vi "RS232test.vi"() -> ()   [LabVIEW 2014]
panel:
  out "Tweet text":string
  in  "Send Tweets?":bool
  out "Run Time (s)":dbl
  out "CTS?":bool
  out "DSR?":bool
  out "Serial Settings:Modem Line Settings:Line DSR State":i16(ring)=-1 items=["Unknown"=-1, "Unasserted"=0, "Asserted"=1]
  out "Serial Settings:Modem Line Settings:Line CTS State":i16(ring)=-1 items=["Unknown"=-1, "Unasserted"=0, "Asserted"=1]
  out "error out":errorcluster
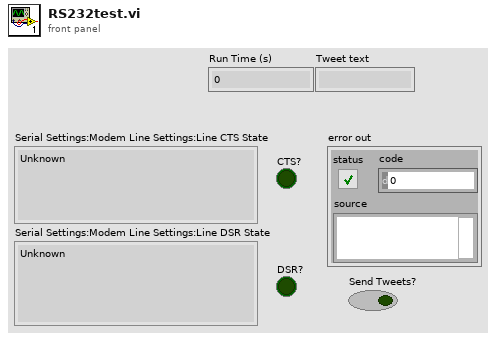
[diagram p1: front panel]
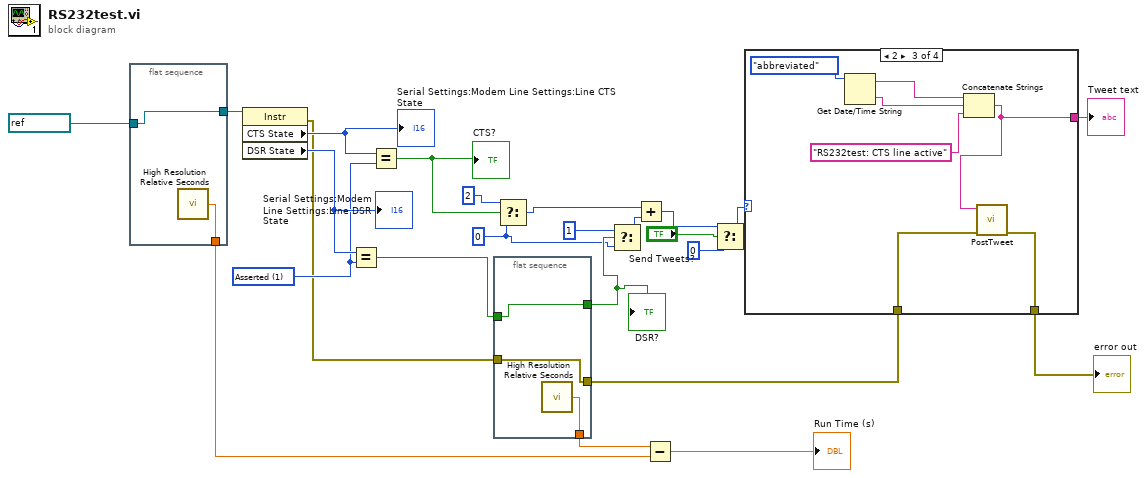
[diagram p0: block diagram]
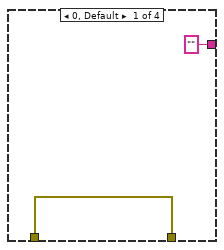
[diagram p2: hidden frame]
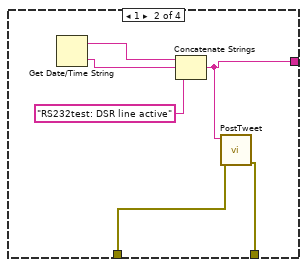
[diagram p3: hidden frame]
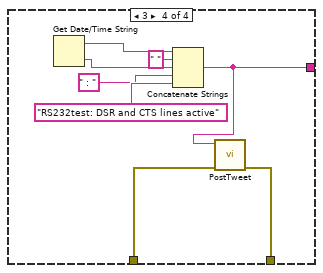
[diagram p4: hidden frame]
diagram:
  w9 = u8 0 ("f")
  w22 = i16 1 items=["Unknown"=-1, "Unasserted"=0, "Asserted"=1] ("Serial Settings:Modem Line Settings:Line DSR State 2")
  n1 = flat-sequence {
    tunnel: refnum<visa-resource-name> "COM1" ("VISA resource name") -> [w26]
    tunnel: [w26] -> w20
    tunnel: [w25] -> w17
    frame #0 {
      n2 = call <vilib>:"High Resolution Relative Seconds.vi"() -> ("relative seconds"=w25:dbl)
    }
  }
  n3 = property class="Instr"(reference=w20) -> (error out=w15:errorcluster, "CTS State"=w23:i16, "DSR State"=w24:i16)  [unwired: 1 in, 1 out]
  "Serial Settings:Modem Line Settings:Line CTS State" <- w23
  "Serial Settings:Modem Line Settings:Line DSR State" <- w24
  n4 = Equal?(x=w24, y=w22) -> (x = y?=w19:bool)
  n5 = Equal?(x=w23, y=w22) -> (x = y?=w12:bool)
  "CTS?" <- w12
  n6 = flat-sequence {
    tunnel: w19 -> [w29]
    tunnel: [w29] -> w10
    tunnel: [w28] -> w18
    tunnel: w15 -> [w27]
    tunnel: [w27] -> w14
    frame #0 {
      n7 = call <vilib>:"High Resolution Relative Seconds.vi"() -> ("relative seconds"=w28:dbl)
    }
  }
  n8 = Select(t=u8 2 ("f"), s=w12, f=w9) -> (s? t:f=w6:u8)
  n9 = Select(t=u8 1 ("f"), s=w10, f=w9) -> (s? t:f=w7:u8)
  n10 = Add(x=w6, y=w7) -> (x+y=w5:u8)
  n11 = Subtract(x=w18, y=w17) -> (x-y=→"Run Time (s)":dbl)
  n12 = Select(t=w5, s="Send Tweets?", f=u8 0) -> (s? t:f=w2:u8)
  n13 = case shown="2" w2 {
    tunnel: w14 -> [w31 w37 w43 w52]
    tunnel: [w31 w36 w44 w51] -> w13
    tunnel: ["" w32 w39 w45] -> w1
    frame 0, Default {
    }
    frame 1 {
      n14 = Get Date/Time String() -> (date string=w35:string, time string=w34:string)  [unwired: 3 in]
      n15 = Concatenate Strings(w35, w34, "RS232test: DSR line active" ("Tweet")) -> (w32:string)
      n16 = call "PostTweet.vi"("error in"=w37, "Tweet"=w32) -> ("error out"=w36:errorcluster)  [unwired: 9 in]
    }
    frame 2 {
      n17 = Get Date/Time String(date format (0)=enum16{"short", "long", "abbreviated"}."abbreviated") -> (date string=w42:string, time string=w41:string)  [unwired: 2 in]
      n18 = Concatenate Strings(w42, w41, "RS232test: CTS line active" ("Tweet")) -> (w39:string)
      n19 = call "PostTweet.vi"("error in"=w43, "Tweet"=w39) -> ("error out"=w44:errorcluster)  [unwired: 9 in]
    }
    frame 3 {
      n20 = Get Date/Time String() -> (date string=w47:string, time string=w50:string)  [unwired: 3 in]
      n21 = Concatenate Strings(w47, " " ("string"), w50, " : " ("string"), "RS232test: DSR and CTS lines active" ("Tweet")) -> (w45:string)
      n22 = call "PostTweet.vi"("error in"=w52, "Tweet"=w45) -> ("error out"=w51:errorcluster)  [unwired: 9 in]
    }
  }
  "error out" <- w13
  "Tweet text" <- w1
  "DSR?" <- w10
